vi "Inventario.vi"(8 "error in (no error)":errorcluster, 10 "Inventario":u16, 11 "Doña Rata Actor in":refnum<class "Doña Rata Actor.lvclass">) -> (0 "error out":errorcluster, 3 "Doña Rata Actor out":refnum<class "Doña Rata Actor.lvclass">)   [LabVIEW 2020, in "Doña Rata Actor.lvlib" / "Doña Rata Actor.lvclass"]
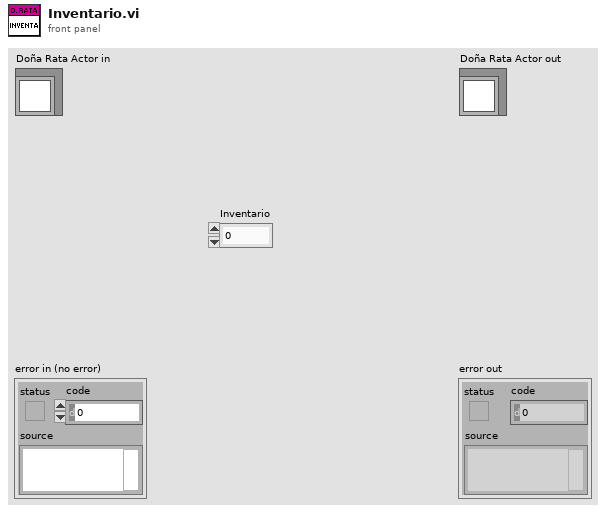
[diagram p1: front panel]
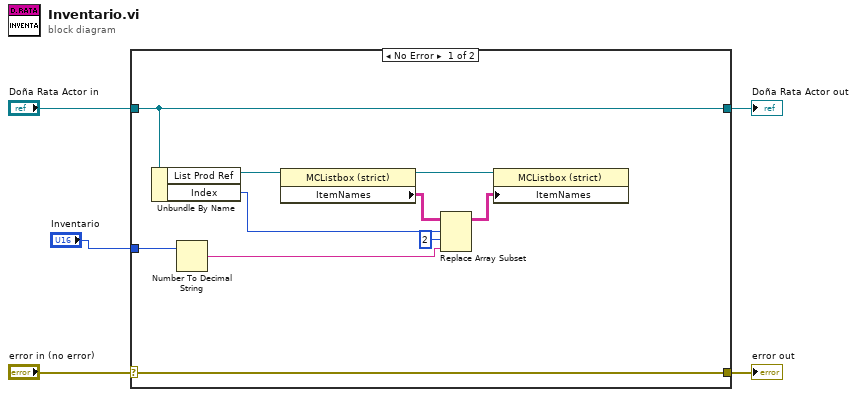
[diagram p0: block diagram]
diagram:
  n1 = case shown="No Error" "error in (no error)" {
    selector: "error in (no error)" -> [w15 w17]
    tunnel: [w15 w17] -> w4
    tunnel: [w14 w16] -> w2
    tunnel: "Doña Rata Actor in" -> [w14 w16]
    tunnel: "Inventario" -> [w13 _]
    frame No Error {
      n2 = Unbundle By Name(w14) -> ("List Prod Ref"=w12:refnum<vi>, "Index"=w8:u16)
      n3 = Number To Decimal String(number=w13) -> (decimal integer string=w6:string)  [unwired: 1 in]
      n4 = property class="MCListbox (strict)"(reference=w12) -> (reference out=w10:refnum<vi>, "ItemNames"=w11:string[][])  [unwired: 1 in, 1 out]
      n5 = Replace Array Subset(array=w11, new element=w6, index (row)=w8, index (col)=2 ("disabled index (col)")) -> (w9:string[][])
      n6 = property class="MCListbox (strict)"(reference=w10, "ItemNames"=w9) -> ()  [unwired: 1 in, 2 out]
    }
    frame Error {
    }
  }
  "error out" <- w4
  "Doña Rata Actor out" <- w2
